vi "WPI_CameraGet Default Frame Rate.vi"() -> (3 "Frame Rate (fps)":T1)   [LabVIEW 2017]
doc: "This software is licensed. Open the labview\\readme\\WPI Robotics Library Open Source License.txt file for more information."
uses:
  <vilib>/Rock Robotics/WPI/Camera/WPI_CameraFrameRate.ctl
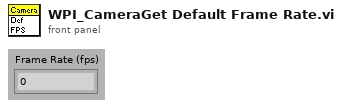
[diagram p1: front panel]
types:
  T1 = typedef "WPI_CameraFrameRate.ctl" = u32
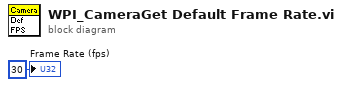
[diagram p0: block diagram]
diagram:
  "Frame Rate (fps)" <- T1 30 ("Frame Rate (fps)")
